vi "F Dwf Digital In Status Data.vi"(8 "error in (no error)":errorcluster, 9 "countOfDataBytes":i32, 10 "rgData":u32, 11 "hdwf":i32) -> (0 "error out":errorcluster, 2 "rgData out":u32, 3 "function return":i32)   [LabVIEW 2019, in "Olasdwf.lvlib"]
doc: "DWFAPI int FDwfDigitalInStatusData(HDWF hdwf, void *rgData, int countOfDataBytes);"
uses:
  Olasdwf.lvlib
  Windows/System32/dwf.dll
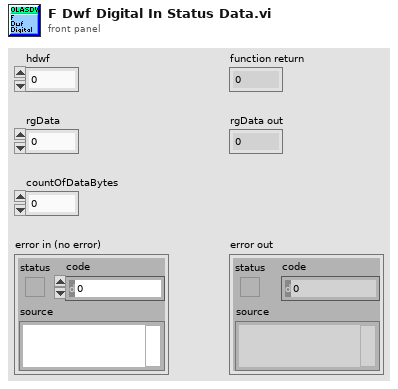
[diagram p1: front panel]
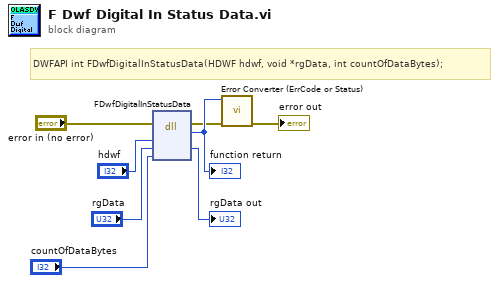
[diagram p0: block diagram]
diagram:
  # "DWFAPI int FDwfDigitalInStatusData(HDWF hdwf, void *rgData, int countOfDataBytes);"
  n1 = dll-call lib="C:/Windows/System32/dwf.*" fn="FDwfDigitalInStatusData"(error in="error in (no error)", "hdwf"="hdwf", "rgData"="rgData", "countOfDataBytes"="countOfDataBytes") -> (error out=w2:errorcluster, w8:i32, "rgData"=→"rgData out":u32)  [unwired: 4 in, 1 out]
  "function return" <- w8
  n2 = call "Error Converter (ErrCode or Status).vi"("error in (no error)"=w2, "error code"=w8) -> ("error out"=→"error out":errorcluster)  [unwired: 9 in]
